vi "ProductBuildingQueryInFunctionToParameters.vi"(11 "ParameterToRead":T1) -> (3 "QueryToRead":string)   [LabVIEW 2014]
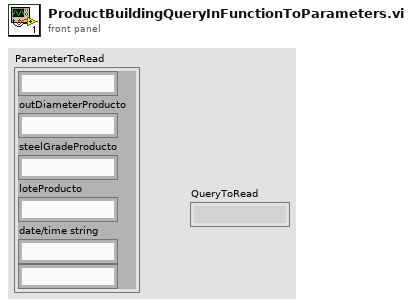
[diagram p1: front panel]
types:
  T1 = cluster{string, "outDiameterProducto":string, "steelGradeProducto":string, "loteProducto":string, "date/time string":string, string}
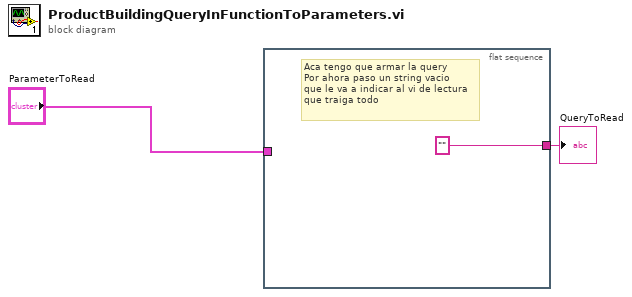
[diagram p0: block diagram]
diagram:
  n1 = flat-sequence {
    tunnel: "ParameterToRead" -> [_]
    tunnel: [""] -> w2
    frame #0 {
      # "Aca tengo que armar la query\nPor ahora paso un string vacio\nque le va a indicar al vi de lectura\nque traiga todo"
    }
  }
  "QueryToRead" <- w2
